vi "Read Attributes.vi"(11 "Return Device Control Msg":refnum<class "Return Device Control Msg.lvclass">) -> (2 "Payload":cluster{"DeviceID":u64, "Control":bool})   [LabVIEW 2016, in "Optimization Framework.lvlib" / "Return Device Control Msg.lvclass"]
uses:
  Return Device Control Msg.lvclass
  Return Device Control Msg.lvclass/Return Device Control Msg.ctl
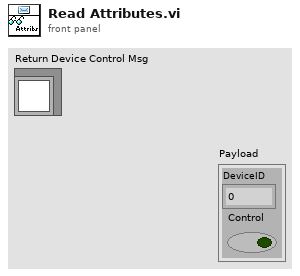
[diagram p1: front panel]
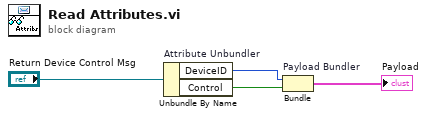
[diagram p0: block diagram]
diagram:
  n1 = Unbundle By Name "Attribute Unbundler"("Return Device Control Msg") -> ("DeviceID"=w2:u64, "Control"=w1:bool)
  n2 = Bundle "Payload Bundler"("DeviceID"=w2, "Control"=w1) -> (→"Payload":cluster{"DeviceID":u64, "Control":bool})  [unwired: 1 in]
